vi "WindowsClusterToSize.vi"(11 "subwindow control 2":T2={"2^n : x"=10, "2^n : y"=10, "lower left box Position"={"X"=1752.0, "Y"=1167.0}, "Height"=0, "Width"=0} {"Width" min=32 max=4704; "Height" min=2 max=3424; "2^n : y" min=1 max=13; "2^n : x" min=1 max=13}) -> (1 "Ny":dbl, 3 "Nx":dbl)   [LabVIEW 2018, in "Photon Filtering.lvlib"]
uses:
  Photon Filtering.lvlib
  <vilib>/Utility/miscctls.llb/LVPointDoubleTypeDef.ctl
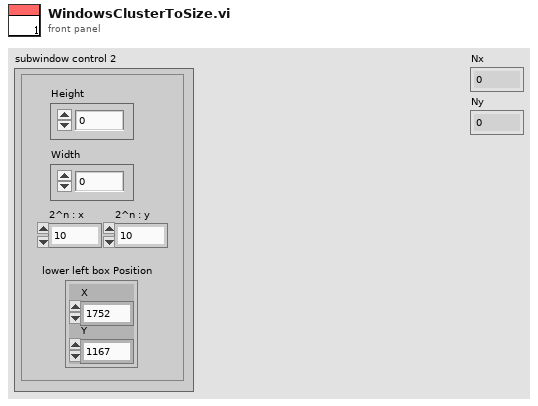
[diagram p1: front panel]
types:
  T1 = typedef "LVPointDoubleTypeDef.ctl" = cluster{"X":dbl, "Y":dbl}
  T2 = cluster{"2^n : x":i8, "2^n : y":i8, "lower left box Position":T1, "Height":i32, "Width":i32}
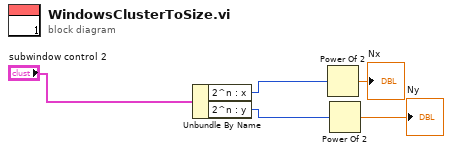
[diagram p0: block diagram]
diagram:
  n1 = Unbundle By Name("subwindow control 2") -> ("2^n : x"=w4:i8, "2^n : y"=w3:i8)
  n2 = Power Of 2(x=w4) -> (2^x=→"Nx":dbl)
  n3 = Power Of 2(x=w3) -> (2^x=→"Ny":dbl)
